vi "Main.vi"() -> ()   [LabVIEW 2016]
doc: "The roboRIO Project template acquires acceleration data from the onboard accelerometer and displays the changes of acceleration values in a waveform chart."
uses:
  <userlib>/ROS for LabVIEW Software/ROS/Code/Console/Servers/ServerSubs/TopicDef.ctl
  <userlib>/ROS for LabVIEW Software/ROS/Code/SubVIs/_ROSDirection.ctl
  <userlib>/ROS for LabVIEW Software/ROS/MessageBuilding/std_msgs/subs/boolScalar.vi
  <userlib>/ROS for LabVIEW Software/ROS/MessageParsing/std_msgs/subs/parse_bool_scalar.vi
panel:
  in  "Boolean":bool
  out "bool":bool
  in  "stop 2":bool
  out "error out 2":errorcluster
  in  "stop":bool
  out "error out":errorcluster
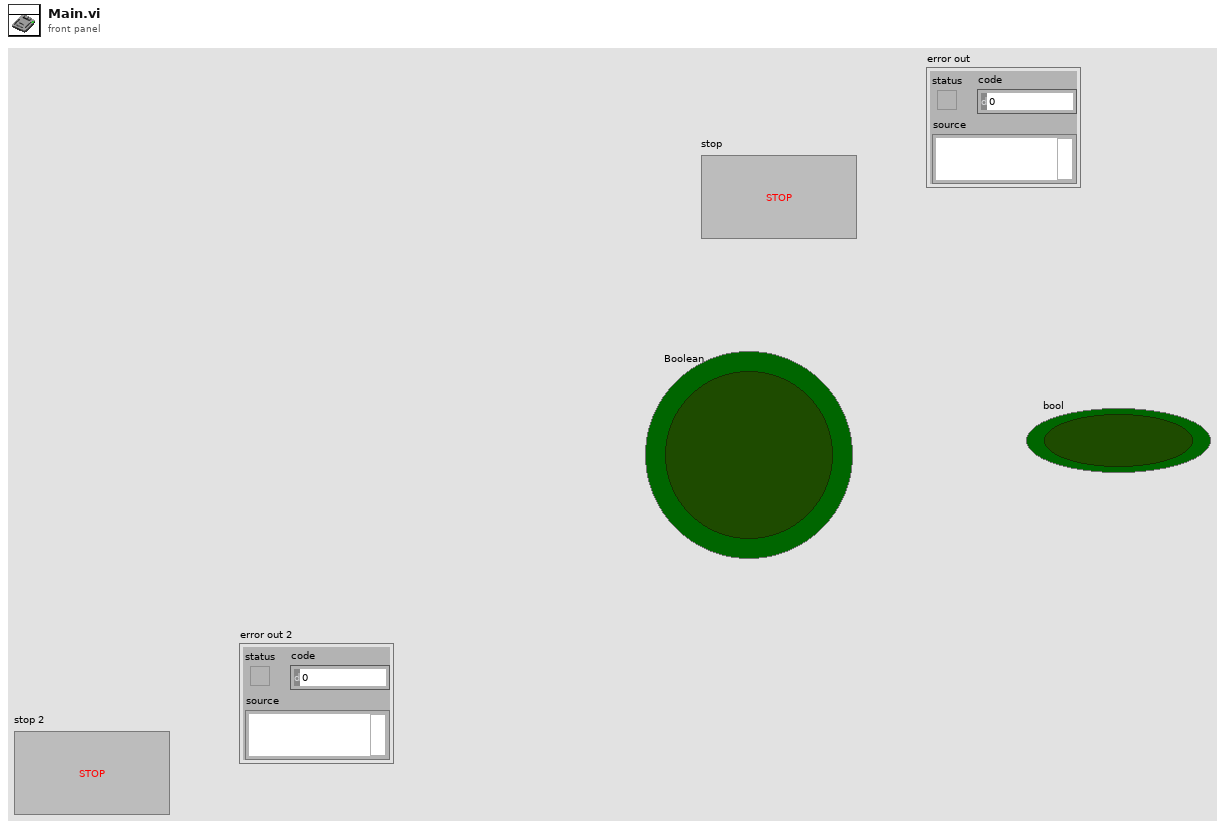
[diagram p1: front panel]
types:
  T1 = typedef "TopicDef.ctl" = cluster{"Topic":string, "Type":string, "Action":T2, "Update (ms)":u16, "queue size":u16}
  T2 = typedef "_ROSDirection.ctl" = enum16{"Node", "Publisher", "Subscriber", "ServiceClient", "ServiceProvider"}
  T3 = typedef "_ROSControl.ctl" = cluster{"topic port":u16, "Node":string, "topic":string, "type":string, "node port":u16, "error ":errorcluster, "Direction":T2, "Update (ms)":u16, "FIFO size":u16}
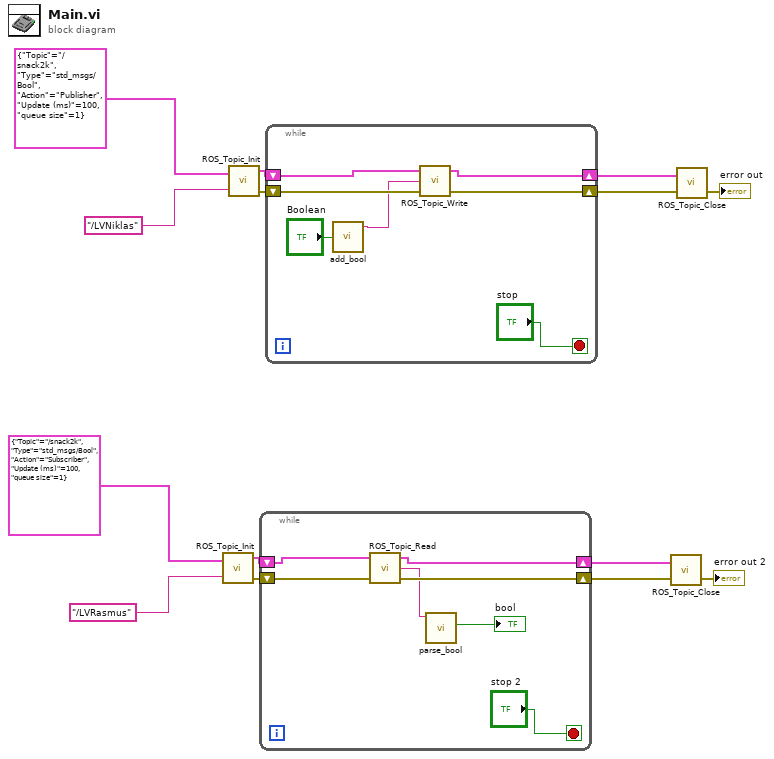
[diagram p0: block diagram]
diagram:
  n1 = call <userlib>:"ROS_Topic_Init.vi"("Definitions"=T1 {"Topic"="/snack2k", "Type"="std_msgs/Bool", "Action"=enum."Subscriber", "Update (ms)"=100, "queue size"=1}, "node"="/LVRasmus") -> ("ROS out"=w3:T3, "error out"=w5:errorcluster)  [unwired: 1 in]
  n2 = call <userlib>:"ROS_Topic_Init.vi"("Definitions"=T1 {"Topic"="/snack2k", "Type"="std_msgs/Bool", "Action"=enum."Publisher", "Update (ms)"=100, "queue size"=1}, "node"="/LVNiklas") -> ("ROS out"=w10:T3, "error out"=w12:errorcluster)  [unwired: 1 in]
  n3 = while {
    shift-right: [w17] -> w4
    shift-left: w5 -> [w19]
    shift-right: [w18] -> w2
    shift-left: w3 -> [w20]
    stop <- "stop 2" stop-if-true
    n4 = call <userlib>:"ROS_Topic_Read.vi"("error in (no error)"=w19, "ROS in"=w20) -> ("error out"=w17:errorcluster, "Reply"=w16:string, "ROS out"=w18:T3)  [unwired: 1 in]
    n5 = call-poly <userlib>:"parse_bool.vi"("msg in"=w16) -> ("bool"=→"bool":bool)  [unwired: 4 in, 2 out]
  }
  n6 = while {
    shift-right: [w27] -> w11
    shift-left: w12 -> [w28]
    shift-right: [w25] -> w9
    shift-left: w10 -> [w26]
    stop <- "stop" stop-if-true
    n7 = call-poly <userlib>:"add_bool.vi"("Boolean"="Boolean") -> ("msg out"=w23:string)  [unwired: 4 in]
    n8 = call <userlib>:"ROS_Topic_Write.vi"("error in (no error)"=w28, "Msg in"=w23, "ROS in"=w26) -> ("error out"=w27:errorcluster, "ROS out"=w25:T3)  [unwired: 1 in]
  }
  n9 = call <userlib>:"ROS_Topic_Close.vi"("error in"=w4, "ROS in"=w2) -> ("error out"=→"error out 2":errorcluster)  [unwired: 2 in]
  n10 = call <userlib>:"ROS_Topic_Close.vi"("error in"=w11, "ROS in"=w9) -> ("error out"=→"error out":errorcluster)  [unwired: 2 in]
